vi "操作日志写入.vi"(8 "error in (no error)":errorcluster, 11 "data in":T1={"时间标识"=timestamp(0 s since 1904-01-01), "参数"="铜", "日志信息"="", "流程参数"=""}) -> (0 "error out":errorcluster)   [LabVIEW 2022 SP3, in "重金属.lvlib"]
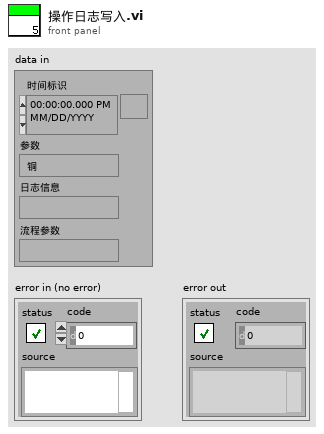
[diagram p1: front panel]
types:
  T1 = cluster{"时间标识":timestamp, "参数":string, "日志信息":string, "流程参数":string}
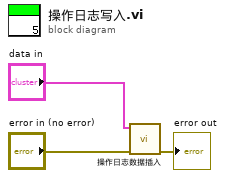
[diagram p0: block diagram]
diagram:
  n1 = call "操作日志数据插入.vi"("data"="data in", "错误输入（无错误）"="error in (no error)") -> ("错误输出"=→"error out":errorcluster)  [unwired: 8 in]
